vi "Disable Lock Plot.vi"(8 "error in (no error)":errorcluster, 9 "Allow Drag":bool, 10 "Plot # Refnum":refnum<vi>, 11 "Locking Refnum":refnum<vi>) -> (0 "error out":errorcluster)   [LabVIEW 2017, in "2D Plot.lvclass"]
uses:
  <vilib>/Math Plots/2D Math Plots/2D Plot/2D Plot/2D Plot.lvclass
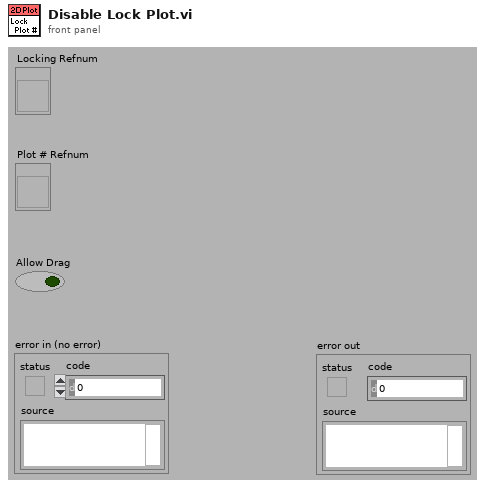
[diagram p1: front panel]
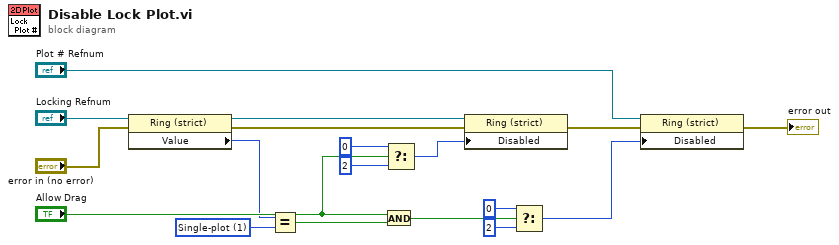
[diagram p0: block diagram]
diagram:
  w11 = 1 items=["Free dragging", "Single-plot", "Multi-plot"] ("Locking")
  n1 = property class="Ring (strict)"(reference="Locking Refnum", error in="error in (no error)") -> (reference out=w4:refnum<vi>, error out=w2:errorcluster, "Value"=w12:i32)
  n2 = Equal?(x=w12, y=w11) -> (x = y?=w17:bool)
  n3 = And(x="Allow Drag", y=w17) -> (x .and. y?=w18:bool)
  n4 = Select(t=u8 0 ("Disabled"), s="Allow Drag", f=u8 2 ("Disabled")) -> (s? t:f=w10:u8)
  n5 = property on="Property Node" class="Ring (strict)"(reference=w4, error in=w2, "Disabled"=w10) -> (error out=w9:errorcluster)  [unwired: 1 out]
  n6 = Select(t=u8 0 ("Disabled"), s=w18, f=u8 2 ("Disabled")) -> (s? t:f=w15:u8)
  n7 = property on="Property Node" class="Ring (strict)"(reference="Plot # Refnum", error in=w9, "Disabled"=w15) -> (error out=→"error out":errorcluster)  [unwired: 1 out]
